vi "Mostly Complete Variant of Brute Force Algorythm.vi"() -> ()   [LabVIEW 2016]
uses:
  Enums/Testing for Desired Points.ctl
  <vilib>/Platform/TimedLoop/XDataNode/timing_clust.ctl
  <vilib>/Platform/TimedLoop/XDataNode/nitl_modes.ctl
  <vilib>/Platform/TimedLoop/XDataNode/wakeup.ctl
  <vilib>/platform/TimedLoop/XDataNode/XDataNode.xnode
  <vilib>/Platform/TimedLoop/XDataNode/XDNodeRunTimeDep.lvlib
panel:
  in  "Array 2":T1[](array[typedef]) items=["Hopper near", "Hopper far", "Peg 1", "Peg 2", "Peg 3", "NT Hopper Near", "NT Hopper Far"]
  in  "Cluster":cluster{dbl, dbl}
  out "array of clusters":cluster{dbl, dbl}[](array[cluster])
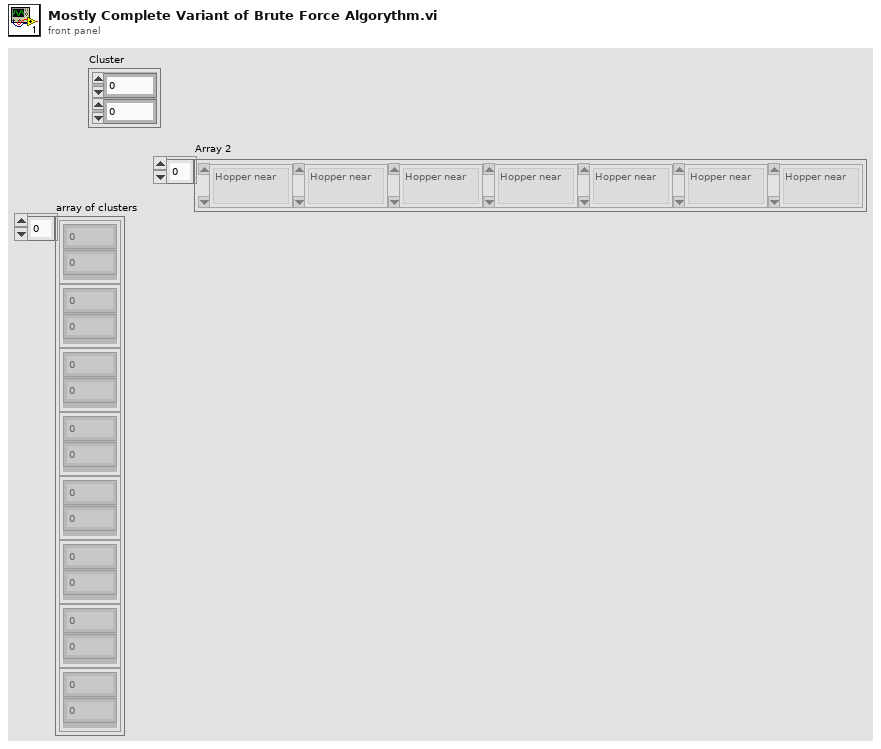
[diagram p1: front panel]
types:
  T1 = typedef "Testing for Desired Points.ctl" = u16
  T2 = typedef "XDNodeRunTimeDep.lvlib/timing_clust.ctl" = cluster{"Expected End [f-1]":u64, "Actual End [f-1]":u64, "Finished Late? [f-1]":bool, "Expected End [i-1]":u64, "Actual End [i-1]":u64, "Finished Late? [i-1]":bool, "Expected Start [i]":u64, "Actual Start [i]":u64, "Expected Start [f]":u64, "Actual Start [f]":u64, "Source Name":string, "Structure Name":string, "Period":i64, "Deadline":i64, "Offset":i64, "Start":i64, "Priority":i32, "Timeout":i32, "Mode":T3, "Wakeup Reason":T4, "Error":errorcluster, "Source Type":string, "Secondary Source Type":string, "Global End Time":u64, "Global Start Time":u64, "Frame Duration":u64, "Iteration Duration":u64, "Assigned CPU":i32, "I/O Scan Engine Mode":u32}
  T3 = typedef "XDNodeRunTimeDep.lvlib/nitl_modes.ctl" = enum32{"No Change", "Process missed periods, maintain original phase", "Discard missed periods, maintain original phase", "Process missed periods, ignore original phase", "Discard missed periods, ignore original phase"}
  T4 = typedef "XDNodeRunTimeDep.lvlib/wakeup.ctl" = enum32{"Normal", "Aborted", "Asynchronous wakeup", "Timing source error", "Timed loop error", "Timeout"}
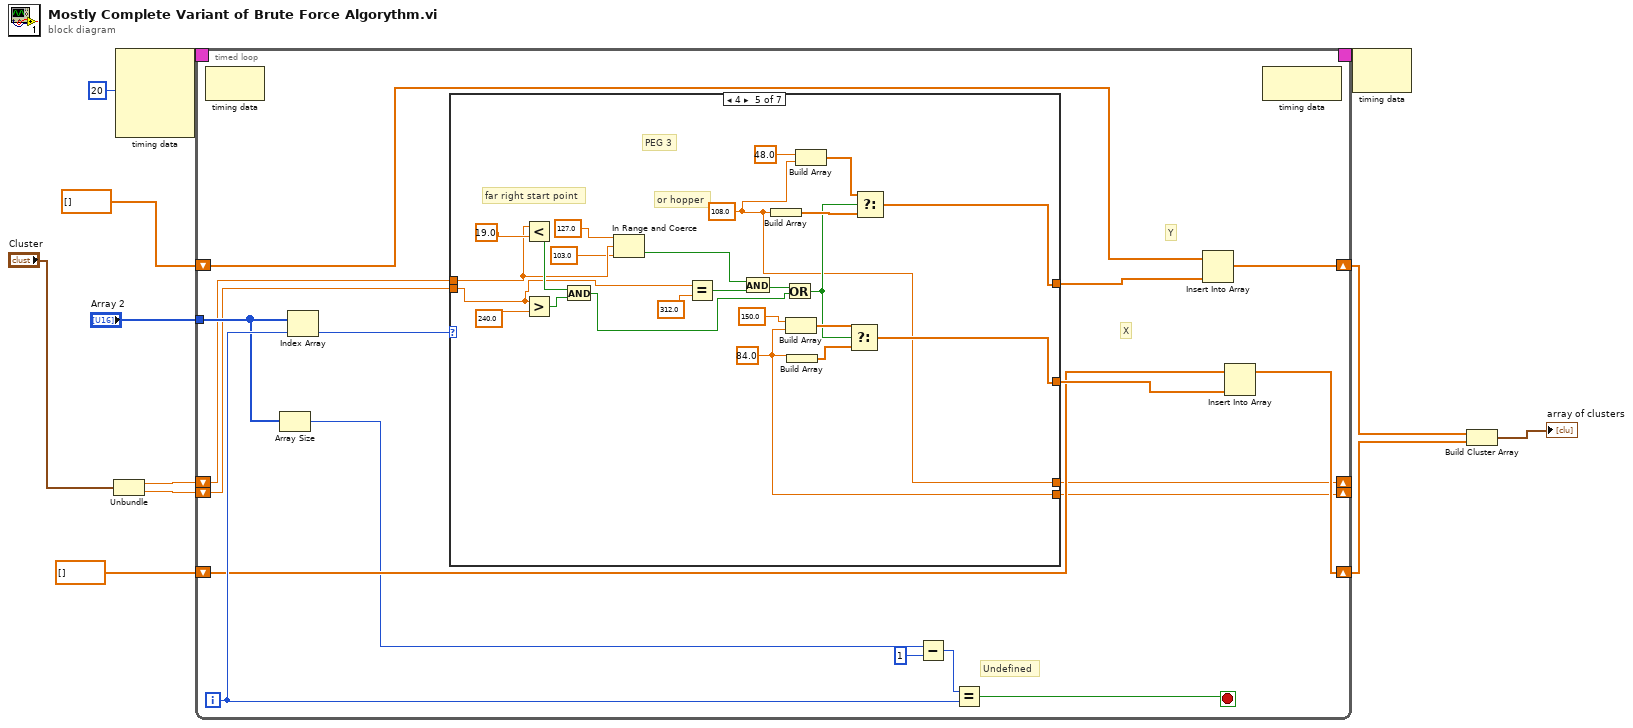
[diagram p0: block diagram]
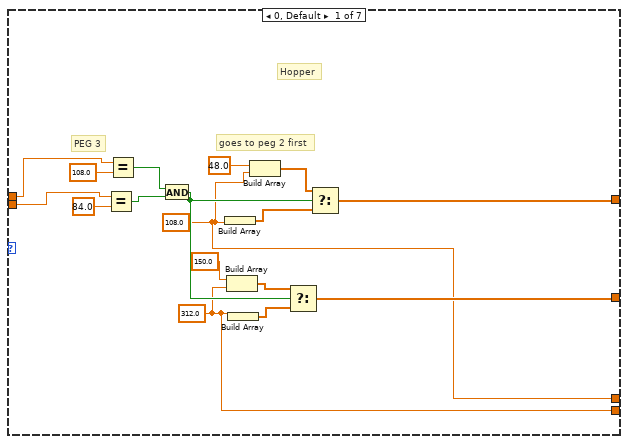
[diagram p2: hidden frame]
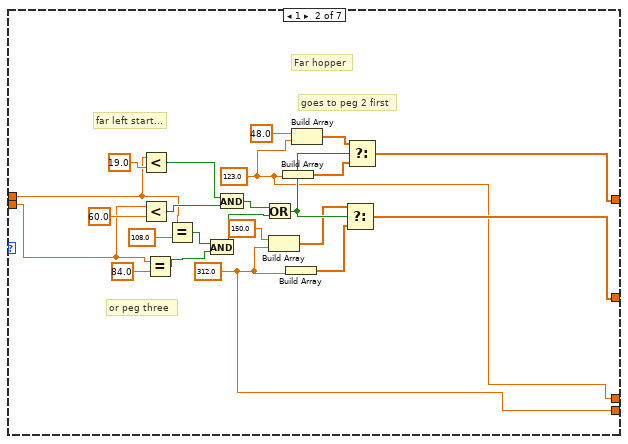
[diagram p3: hidden frame]
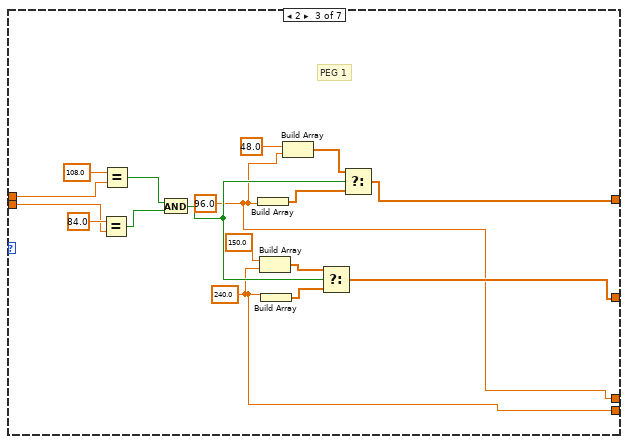
[diagram p4: hidden frame]
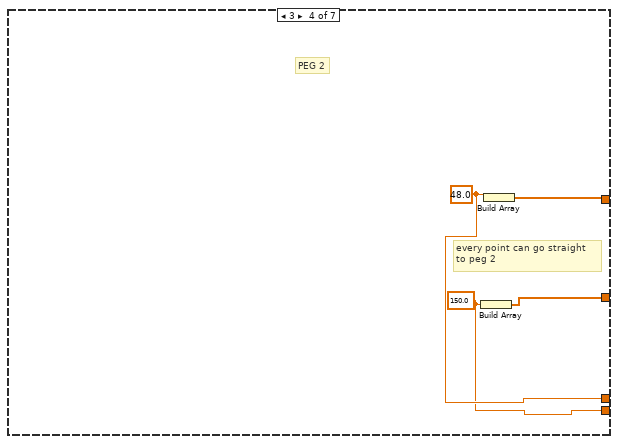
[diagram p5: hidden frame]
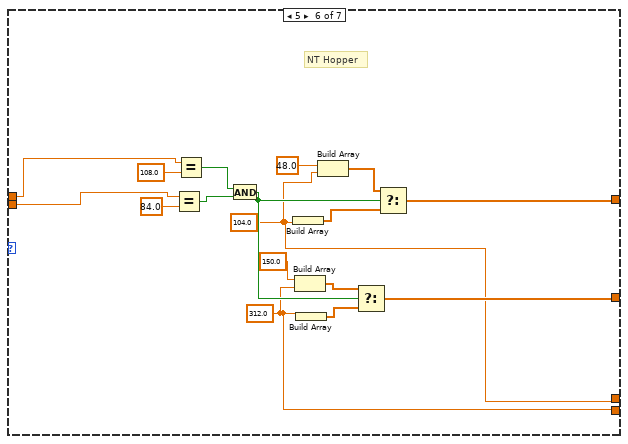
[diagram p6: hidden frame]
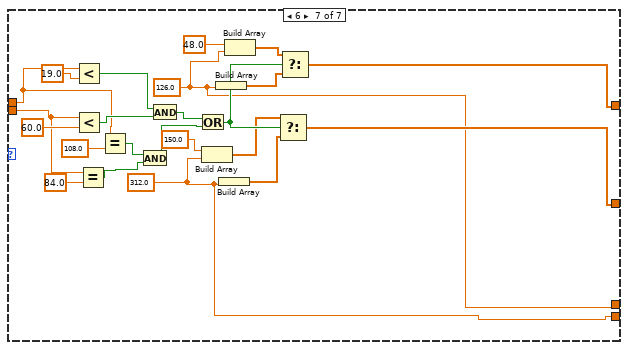
[diagram p7: hidden frame]
diagram:
  n1 = Unbundle("Cluster") -> (w4:dbl, w3:dbl)
  n2 = node-c288(i64 20 ("Period")) -> (w12:T2)  [unwired: 3 in]
  n3 = timed-loop "Timed Loop" {
    tunnel: "Array 2" -> [w20]
    timing: w12 -> [_]
    timing-out: [_] -> w11
    shift-right: [w21] -> w7
    shift-left: dbl[] [] -> [w25]
    shift-right: [w24] -> w6
    shift-left: dbl[] [] -> [w22]
    shift-right: [w16] -> _
    shift-left: w3 -> [w13]
    shift-right: [w15] -> _
    shift-left: w4 -> [w14]
    i -> [w27]
    stop <- w28 stop-if-true
    # "X"
    # "Y"
    # "Undefined"
    n4 = node-c288() -> ()  [unwired: 1 in, 1 out]
    n5 = Array Size(array=w20) -> (size(s)=w19:i32)
    n6 = Index Array(array=w20, index=w27) -> (element=w29:T1)
    n7 = case shown="4" w29 {
      tunnel: [w44 w54 w82 w91 w108 w122 w145] -> w26
      tunnel: [w42 w53 w81 w92 w107 w121 w144] -> w23
      tunnel: w14 -> [w34 w52 w74 _ w98 w119 w137]
      tunnel: w13 -> [w35 w51 w75 _ w95 w120 w136]
      tunnel: [w33 w49 w72 w89 w96 w117 w134] -> w16
      tunnel: [w32 w50 w73 w90 w97 w118 w135] -> w15
      frame 0, Default {
        w33 = 312.0
        w32 = 108.0
        # "goes to peg 2 first"
        # "PEG 3"
        # "Hopper"
        n8 = Equal?(x=w35, y=84.0) -> (x = y?=w45:bool)
        n9 = Equal?(x=w34, y=108.0) -> (x = y?=w46:bool)
        n10 = And(x=w46, y=w45) -> (x .and. y?=w43:bool)
        n11 = Build Array(w32) -> (w37:dbl[])
        n12 = Build Array(150.0, w33) -> (w40:dbl[])
        n13 = Build Array(w33) -> (w39:dbl[])
        n14 = Build Array(48.0, w32) -> (w36:dbl[])
        n15 = Select(t=w40, s=w43, f=w39) -> (s? t:f=w42:dbl[])
        n16 = Select(t=w36, s=w43, f=w37) -> (s? t:f=w44:dbl[])
      }
      frame 1 {
        w49 = 312.0
        w50 = 123.0
        # "Far hopper"
        # "goes to peg 2 first"
        # "or peg three"
        # "far left start..."
        n17 = Less?(x=w52, y=19.0) -> (x < y?=w68:bool)
        n18 = Less?(x=w51, y=60.0) -> (x < y?=w69:bool)
        n19 = Equal?(x=w51, y=84.0) -> (x = y?=w57:bool)
        n20 = Equal?(x=w52, y=108.0) -> (x = y?=w58:bool)
        n21 = And(x=w58, y=w57) -> (x .and. y?=w56:bool)
        n22 = And(x=w68, y=w69) -> (x .and. y?=w67:bool)
        n23 = Or(x=w67, y=w56) -> (x .or. y?=w66:bool)
        n24 = Build Array(150.0, w49) -> (w63:dbl[])
        n25 = Build Array(w50) -> (w55:dbl[])
        n26 = Build Array(w49) -> (w62:dbl[])
        n27 = Build Array(48.0, w50) -> (w61:dbl[])
        n28 = Select(t=w63, s=w66, f=w62) -> (s? t:f=w53:dbl[])
        n29 = Select(t=w61, s=w66, f=w55) -> (s? t:f=w54:dbl[])
      }
      frame 2 {
        w72 = 240.0
        w73 = 96.0
        # "PEG 1"
        n30 = Equal?(x=84.0, y=w75) -> (x = y?=w77:bool)
        n31 = Equal?(x=108.0, y=w74) -> (x = y?=w78:bool)
        n32 = And(x=w78, y=w77) -> (x .and. y?=w76:bool)
        n33 = Build Array(w73) -> (w84:dbl[])
        n34 = Build Array(150.0, w72) -> (w87:dbl[])
        n35 = Build Array(w72) -> (w86:dbl[])
        n36 = Build Array(48.0, w73) -> (w83:dbl[])
        n37 = Select(t=w87, s=w76, f=w86) -> (s? t:f=w81:dbl[])
        n38 = Select(t=w83, s=w76, f=w84) -> (s? t:f=w82:dbl[])
      }
      frame 3 {
        w89 = 150.0
        w90 = 48.0
        # "every point can go straight \nto peg 2"
        # "PEG 2"
        n39 = Build Array(w89) -> (w92:dbl[])
        n40 = Build Array(w90) -> (w91:dbl[])
      }
      frame 4 {
        w96 = 84.0
        w97 = 108.0
        # "PEG 3"
        # "or hopper"
        # "far right start point"
        n41 = Less?(x=w98, y=19.0) -> (x < y?=w103:bool)
        n42 = Greater?(x=w95, y=240.0) -> (0:w104:bool)
        n43 = And(x=w103, y=w104) -> (x .and. y?=w102:bool)
        n44 = In Range and Coerce(upper limit=127.0, x=w98, lower limit=103.0) -> (In Range?=w99:bool)  [unwired: 1 out]
        n45 = Equal?(x=w95, y=312.0) -> (x = y?=w115:bool)
        n46 = And(x=w99, y=w115) -> (x .and. y?=w101:bool)
        n47 = Build Array(w97) -> (w109:dbl[])
        n48 = Or(x=w101, y=w102) -> (x .or. y?=w100:bool)
        n49 = Build Array(150.0, w96) -> (w112:dbl[])
        n50 = Build Array(w96) -> (w111:dbl[])
        n51 = Build Array(48.0, w97) -> (w110:dbl[])
        n52 = Select(t=w112, s=w100, f=w111) -> (s? t:f=w107:dbl[])
        n53 = Select(t=w110, s=w100, f=w109) -> (s? t:f=w108:dbl[])
      }
      frame 5 {
        w117 = 312.0
        w118 = 104.0
        # "NT Hopper"
        n54 = Equal?(x=w120, y=84.0) -> (x = y?=w126:bool)
        n55 = Equal?(x=w119, y=108.0) -> (x = y?=w125:bool)
        n56 = And(x=w125, y=w126) -> (x .and. y?=w127:bool)
        n57 = Build Array(w118) -> (w132:dbl[])
        n58 = Build Array(150.0, w117) -> (w129:dbl[])
        n59 = Build Array(w117) -> (w130:dbl[])
        n60 = Build Array(48.0, w118) -> (w133:dbl[])
        n61 = Select(t=w129, s=w127, f=w130) -> (s? t:f=w121:dbl[])
        n62 = Select(t=w133, s=w127, f=w132) -> (s? t:f=w122:dbl[])
      }
      frame 6 {
        w134 = 312.0
        w135 = 126.0
        n63 = Less?(x=w137, y=19.0) -> (x < y?=w153:bool)
        n64 = Less?(x=w136, y=60.0) -> (x < y?=w154:bool)
        n65 = Equal?(x=w136, y=84.0) -> (x = y?=w140:bool)
        n66 = Equal?(x=w137, y=108.0) -> (x = y?=w141:bool)
        n67 = And(x=w141, y=w140) -> (x .and. y?=w139:bool)
        n68 = And(x=w153, y=w154) -> (x .and. y?=w152:bool)
        n69 = Or(x=w152, y=w139) -> (x .or. y?=w151:bool)
        n70 = Build Array(150.0, w134) -> (w148:dbl[])
        n71 = Build Array(w135) -> (w138:dbl[])
        n72 = Build Array(w134) -> (w147:dbl[])
        n73 = Build Array(48.0, w135) -> (w146:dbl[])
        n74 = Select(t=w148, s=w151, f=w147) -> (s? t:f=w144:dbl[])
        n75 = Select(t=w146, s=w151, f=w138) -> (s? t:f=w145:dbl[])
      }
    }
    n76 = Subtract(x=w19, y=1) -> (x-y=w17:i32)
    n77 = Equal?(x=w17, y=w27) -> (x = y?=w28:bool)
    n78 = Insert Into Array(array=w25, new element=w26) -> (w21:dbl[])  [unwired: 1 in]
    n79 = Insert Into Array(array=w22, new element=w23) -> (w24:dbl[])  [unwired: 1 in]
    n80 = node-c288() -> ()  [unwired: 1 in, 1 out]
  }
  n81 = node-c288(w11) -> ()  [unwired: 1 out]
  n82 = Build Cluster Array(w7, w6) -> (→"array of clusters":cluster{dbl, dbl}[])
